vi "MakeHTMLHeader.vi"(3 "Escape Contents":bool, 4 "Header Content":string, 5 "Header Type":enum16{"h1", "h2", "h3", "h4", "h5", "h6"}(ring)) -> (1 "Header Element":string)   [LabVIEW 2018, in "ArgosLib.lvlib"]
uses:
  ArgosLib.lvlib
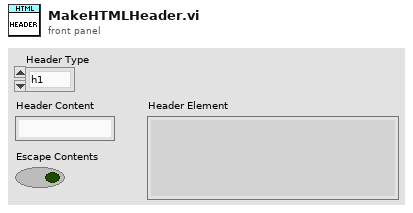
[diagram p1: front panel]
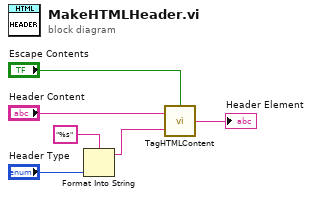
[diagram p0: block diagram]
diagram:
  n1 = Format Into String(format string="%s", "Header Type") -> (resulting string=w1:string)  [unwired: 2 in, 1 out]
  n2 = call "TagHTMLContent.vi"("Escape Contents"="Escape Contents", "Tag"=w1, "Element Contents"="Header Content") -> ("Tagged Contents"=→"Header Element":string)
